vi "FTW-Test-Socket-Stress-PubSub.vi"() -> (0 "Test Result":errorcluster)   [LabVIEW 2014]
panel:
  in  "Test to Perform":T1(radio)=enum."12x100x10k"
  out "Progress":dbl(slide) scale=0.0..1.0
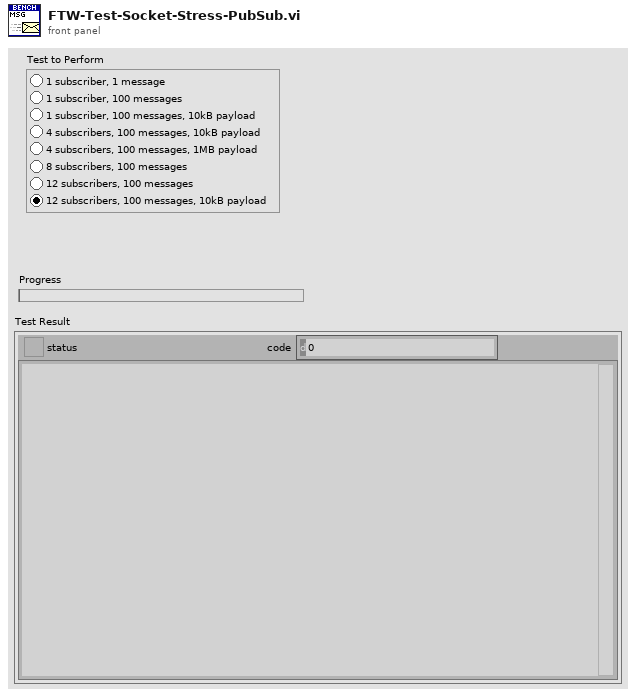
[diagram p1: front panel]
types:
  T1 = enum32{"1x1x0", "1x100x0", "1x100x10k", "4x100x10k", "4x100x1M", "8x100x0", "12x100x0", "12x100x10k"}
  T2 = typedef "FTW-Socket-Core-TransportScheme.ctl" = enum16{"TCP (tcp://)", "Inter-Process (ipc://)", "In-Process (inproc://)", "WebSocket (ws://)"}
  T3 = cluster{i32, "Bytes Recv'd":i32, "Messages Recv'd":i32}
  T4 = typedef "FTW-ERR-ExceptionType.ctl" = enum16{"OK", "Info", "Warning", "Error"}
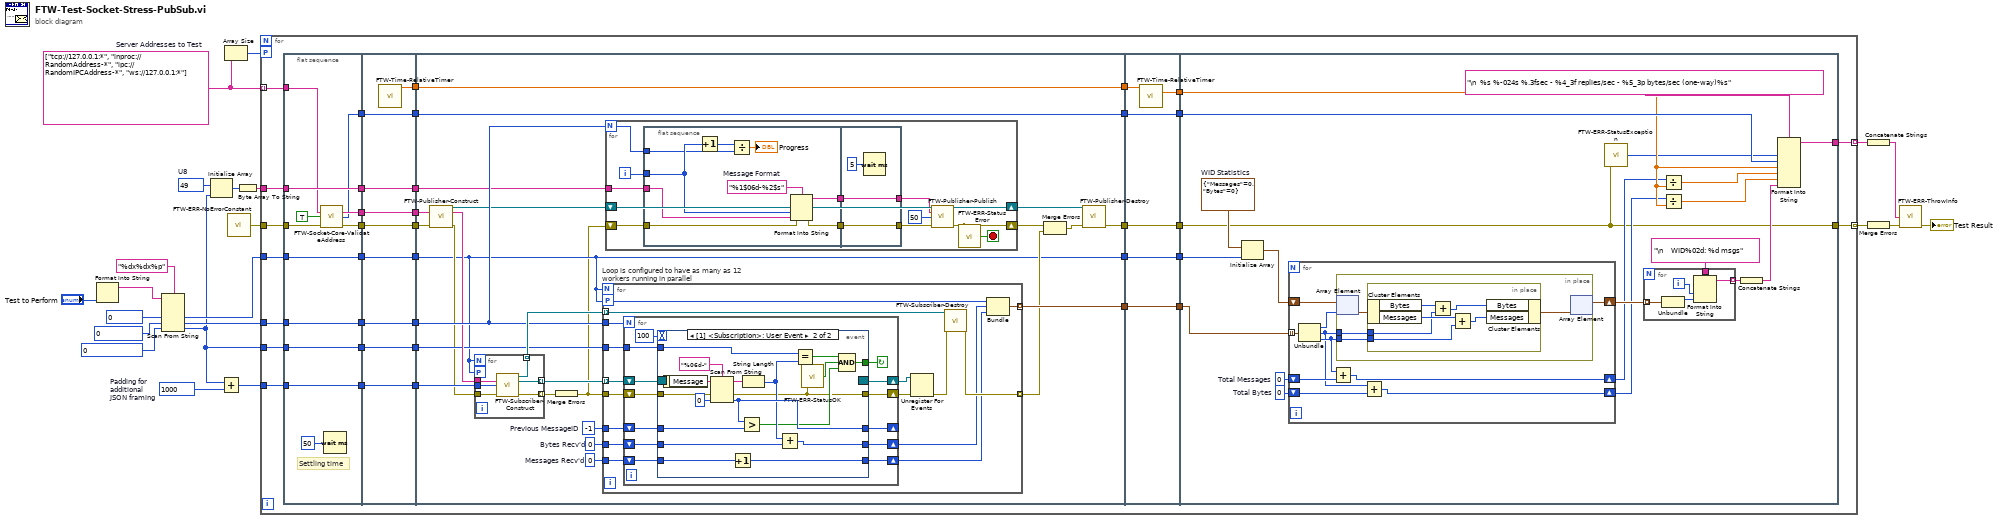
[diagram p0: block diagram]
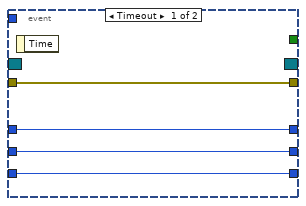
[diagram p2: hidden frame]
diagram:
  w2 = string[] ["tcp://127.0.0.1:*", "inproc://RandomAddress-*", "ipc://RandomIPCAddress-*", "ws://127.0.0.1:*"]  # Server Addresses to Test
  w19 = 1000  # Padding for additional JSON framing
  w22 = u8 49  # U8
  n1 = Format Into String("Test to Perform") -> (resulting string=w12:string)  [unwired: 3 in, 1 out]
  n2 = Scan From String(format string="%dx%dx%p", input string=w12, default 1=0, default 2=0, default 3=0) -> (output 1=w11:i32, output 2=w10:i32, output 3=w1:i32)  [unwired: 2 in, 3 out]
  n3 = Initialize Array(w22, w1) -> (w21:u8[])
  n4 = Add(x=w1, y=w19) -> (x+y=w18:i32)
  n5 = Array Size(array=w2) -> (size(s)=w3:i32)
  n6 = call "FTW-ERR-NoErrorConstant.vi"() -> ("no error"=w4:errorcluster)
  n7 = Byte Array To String(unsigned byte array=w21) -> (string=w20:string)
  n8 = for {
    tunnel: w2 -> [w51] mode=indexing
    tunnel: w11 -> [w50]
    tunnel: w10 -> [w48]
    tunnel: w4 -> [w47]
    tunnel: w20 -> [w40]
    tunnel: w18 -> [w34]
    tunnel: [w33] -> w9 mode=indexing
    tunnel: [w32] -> w7 mode=indexing
    workers-P: w3 -> [_]
    tunnel: w1 -> [w23]
    n9 = flat-sequence {
      tunnel: [w61] -> w58
      tunnel: [w63] -> w52
      tunnel: w47 -> [w62]
      tunnel: w48 -> [w67]
      tunnel: w50 -> [w68]
      tunnel: w51 -> [w64]
      tunnel: [w68] -> w45
      tunnel: [w67] -> w43
      tunnel: [w69] -> w41
      tunnel: w40 -> [w69]
      tunnel: [w66] -> w35
      tunnel: w34 -> [w66]
      tunnel: [w60] -> w30
      tunnel: [w59] -> w24
      tunnel: w23 -> [w59]
      tunnel: [w79] -> w57
      tunnel: [w74] -> w56
      tunnel: w58 -> [w79]
      tunnel: [w78] -> w53
      tunnel: w52 -> [w78]
      tunnel: [w77] -> w46
      tunnel: w45 -> [w77]
      tunnel: [w76] -> w44
      tunnel: w43 -> [w76]
      tunnel: [w75] -> w42
      tunnel: w41 -> [w75]
      tunnel: [w73] -> w36
      tunnel: w35 -> [w73]
      tunnel: [w72] -> w31
      tunnel: w30 -> [w72]
      tunnel: [w71] -> w25
      tunnel: w24 -> [w71]
      tunnel: [w93] -> w55
      tunnel: [w104] -> w54
      tunnel: [w103] -> w49
      tunnel: w44 -> [w96]
      tunnel: w46 -> [w81]
      tunnel: w57 -> [w102]
      tunnel: w56 -> [w104]
      tunnel: w53 -> [w92]
      tunnel: w42 -> [w88]
      tunnel: w36 -> [w89]
      tunnel: w31 -> [w87]
      tunnel: [w87] -> w28
      tunnel: [w81] -> w26
      tunnel: w25 -> [w83]
      tunnel: w55 -> [w192]
      tunnel: w54 -> [w190]
      tunnel: w49 -> [w191]
      tunnel: [w192] -> w39
      tunnel: [w189] -> w38
      tunnel: [w191] -> w37
      tunnel: [w188] -> w29
      tunnel: w28 -> [w188]
      tunnel: [w187] -> w27
      tunnel: w26 -> [w187]
      tunnel: w39 -> [w193]
      tunnel: w38 -> [w209]
      tunnel: w37 -> [w206]
      tunnel: [w193] -> w33
      tunnel: [w211] -> w32
      tunnel: w29 -> [w210]
      tunnel: w27 -> [w204]
      frame #0 {
        # "Settling time"
        n10 = call "FTW-Socket-Core-ValidateAddress.vi"("Address"=w64, "Allow wildcard replacement?"=TRUE, "error in"=w62) -> ("Sanitized Address"=w63:string, "Message Transport Scheme"=w60:T2, "error out"=w61:errorcluster)  [unwired: 10 in]
        n11 = Wait (ms)(milliseconds to wait=u32 50) -> ()  [unwired: 1 out]
      }
      frame #1 {
        n12 = call "FTW-Time-RelativeTimer.vi"() -> ("Current Uptime"=w74:dbl)  [unwired: 13 in, 2 out]
      }
      frame #2 {
        w84 = 0  # Messages Recv'd
        w86 = -1  # Previous MessageID
        w85 = 0  # Bytes Recv'd
        n13 = call "FTW-Publisher-Construct.vi"("Instance Inbox Address"=w92, "error in"=w102) -> ("FTW Publisher"=w91:refnum<data-value>, "Resolved Inbox Address"=w90:string, "error out"=w82:errorcluster)  [unwired: 11 in]
        n14 = for {
          N: w81 -> [_]
          workers-P: w81 -> [_]
          tunnel: w90 -> [w110]
          tunnel: w82 -> [w109]
          tunnel: [w108] -> w98 mode=indexing
          tunnel: [w107] -> w97 mode=indexing
          tunnel: [w106] -> w100 mode=indexing
          tunnel: w89 -> [w105]
          n15 = call "FTW-Subscriber-Construct.vi"("Publisher Address"=w110, "Receive Message Size Limit"=w105, "error in"=w109) -> ("FTW Subscriber"=w108:refnum<data-value>, "Subscription"=w107:refnum<event-registration>, "error out"=w106:errorcluster)  [unwired: 10 in]
        }
        n16 = Merge Errors(w100) -> (w80:errorcluster)
        n17 = for "Loop is configured to have as many as 12 workers running in parallel" {
          N: w81 -> [_]
          workers-P: w81 -> [w147]
          tunnel: [w151] -> w103 mode=indexing
          tunnel: [w146] -> w101 mode=indexing
          tunnel: w98 -> [w148] mode=indexing
          tunnel: w97 -> [w150] mode=indexing
          tunnel: w96 -> [w145]
          tunnel: w80 -> [w138]
          tunnel: w83 -> [w141]
          tunnel: w86 -> [w140]
          tunnel: w85 -> [w139]
          tunnel: w84 -> [w137]
          n18 = for {
            N: w145 -> [_]
            shift-right: [w162] -> w149
            shift-left: w150 -> [w164]
            shift-right: [w161] -> w144
            shift-left: w138 -> [w163]
            shift-right: [w156] -> w142
            shift-left: w139 -> [w158]
            shift-right: [w157] -> _
            shift-left: w140 -> [w159]
            tunnel: w141 -> [w160]
            shift-right: [w154] -> w136
            shift-left: w137 -> [w155]
            stop <- w153 continue-if-true
            n19 = event shown="[1] <Subscription>: User Event" {
              selector: w164 -> [_ _]
              dyn-events: [_ _] -> w162
              timeout: 100 -> [_ _]
              tunnel: [_ w171] -> w153
              tunnel: [w168 w172] -> w161
              tunnel: w163 -> [w168 w184]
              tunnel: w160 -> [_ w185]
              tunnel: w159 -> [w167 w182]
              tunnel: w158 -> [w166 w183]
              tunnel: [w167 w181] -> w157
              tunnel: [w166 w177] -> w156
              tunnel: w155 -> [w165 w178]
              tunnel: [w165 w176] -> w154
              event Timeout {
                n20 = event-data() -> ()  [unwired: 1 in, 1 out]
              }
              event User Event {
                n21 = event-data() -> ("Message"=w170:string)  [unwired: 1 in]
                n22 = Scan From String(format string="%06d-", input string=w170, error in=w184, default 1=0 ("default value 1")) -> (remaining string=w169:string, error out=w172:errorcluster, output 1=w181:i32)  [unwired: 1 in, 1 out]
                n23 = Increment(x=w178) -> (x+1=w176:i32)
                n24 = Greater?(x=w181, y=w182) -> (0:w174:bool)
                n25 = String Length(string=w169) -> (length=w179:i32)
                n26 = Add(x=w179, y=w183) -> (x+y=w177:i32)
                n27 = Equal?(x=w185, y=w179) -> (x = y?=w175:bool)
                n28 = call "FTW-ERR-StatusOK.vi"("error to check"=w172) -> ("Status OK?"=w173:bool)
                n29 = Compound Arithmetic op=AND(w175, w173, w174) -> (w171:bool)
              }
            }
          }
          n30 = Unregister For Events(event registration refnum=w149, error in=w144) -> (error out=w143:errorcluster)
          n31 = call "FTW-Subscriber-Destroy.vi"("FTW Subscriber"=w148, "error in"=w143) -> ("error out"=w146:errorcluster)  [unwired: 13 in]
          n32 = Bundle(w147, "Bytes Recv'd"=w142, "Messages Recv'd"=w136) -> (w151:T3)  [unwired: 1 in]
        }
        n33 = for {
          N: w96 -> [w113]
          shift-right: [w122] -> w99
          shift-left: w91 -> [w123]
          tunnel: w88 -> [w115]
          shift-right: [w120] -> w95
          shift-left: w80 -> [w117]
          i -> [w114]
          stop <- w119 stop-if-true
          n34 = flat-sequence {
            tunnel: w117 -> [w132]
            tunnel: [w131] -> w116
            tunnel: w115 -> [w130]
            tunnel: w114 -> [w126]
            tunnel: w113 -> [w125]
            tunnel: [w124] -> w111
            tunnel: [w135] -> w118
            tunnel: w116 -> [w135]
            tunnel: [w133] -> w112
            tunnel: w111 -> [w133]
            frame #0 {
              w129 = "%1$06d-%2$s"  # Message Format
              n35 = Increment(x=w126) -> (x+1=w127:i32)
              n36 = Divide(x=w127, y=w125) -> (x/y=→"Progress":dbl)
              n37 = Format Into String(format string=w129, error in=w132, w126, w130) -> (resulting string=w124:string, error out=w131:errorcluster)  [unwired: 1 in]
            }
            frame #1 {
              n38 = Wait (ms)(milliseconds to wait=u32 5) -> ()  [unwired: 1 out]
            }
          }
          n39 = call "FTW-Publisher-Publish.vi"("FTW Publisher"=w123, "Message"=w112, "Send Timeout"=50, "error in"=w118) -> ("FTW Publisher out"=w122:refnum<data-value>, "error out"=w120:errorcluster)  [unwired: 10 in]
          n40 = call "FTW-ERR-StatusError.vi"("error to check"=w120) -> ("Error?"=w119:bool)
        }
        n41 = Merge Errors(w95, w101) -> (w94:errorcluster)
        n42 = call "FTW-Publisher-Destroy.vi"("FTW Publisher"=w99, "error in"=w94) -> ("error out"=w93:errorcluster)  [unwired: 13 in]
      }
      frame #3 {
        n43 = call "FTW-Time-RelativeTimer.vi"("Previous Uptime"=w190) -> ("Elapsed Time"=w189:dbl)  [unwired: 12 in, 2 out]
      }
      frame #4 {
        w198 = 0  # Total Messages
        w197 = 0  # Total Bytes
        w205 = cluster{"Messages":i32, "Bytes":i32} {"Messages"=0, "Bytes"=0}  # WID Statistics
        n44 = Initialize Array(w205, w204) -> (w203:cluster{"Messages":i32, "Bytes":i32}[])
        n45 = for {
          tunnel: w206 -> [w227] mode=indexing
          shift-right: [w224] -> w202
          shift-left: w203 -> [w226]
          shift-right: [w220] -> w196
          shift-left: w198 -> [w223]
          shift-right: [w221] -> w195
          shift-left: w197 -> [w222]
          n46 = Unbundle(w227) -> (w225:i32, "Bytes Recv'd"=w218:i32, "Messages Recv'd"=w219:i32)
          n47 = Add(x=w219, y=w223) -> (x+y=w220:i32)
          n48 = in-place {
            in-place-border: w218 -> [w230]
            in-place-border: w219 -> [w229]
            n49 = in-place-array #1(w226, w225) -> (w231:cluster{"Messages":i32, "Bytes":i32})
            n50 = in-place {
              in-place-border: w230 -> [w233]
              in-place-border: w229 -> [w232]
              n51 = in-place-cluster #2(w231) -> ("Bytes"=w237:i32, "Messages"=w235:i32)
              n52 = Add(x=w237, y=w233) -> (x+y=w236:i32)
              n53 = Add(x=w235, y=w232) -> (x+y=w234:i32)
              n54 = in-place-cluster #2("Bytes"=w236, "Messages"=w234) -> (w228:cluster{"Messages":i32, "Bytes":i32})
            }
            n55 = in-place-array #1(w228) -> (w224:cluster{"Messages":i32, "Bytes":i32}[])  [unwired: 1 out]
          }
          n56 = Add(x=w218, y=w222) -> (x+y=w221:i32)
        }
        n57 = call "FTW-ERR-StatusException.vi"("error to check"=w193) -> ("Exception"=w194:T4)
        n58 = for {
          tunnel: w202 -> [w217] mode=indexing
          tunnel: [w215] -> w201 mode=indexing
          tunnel: "\n    WID%02d: %d msgs" ("format string") -> [w214]
          i -> [w216]
          n59 = Unbundle(w217) -> ("Messages"=w213:i32)  [unwired: 1 out]
          n60 = Format Into String(format string=w214, w216, w213) -> (resulting string=w215:string)  [unwired: 2 in, 1 out]
        }
        n61 = Divide(x=w196, y=w209) -> (x/y=w208:dbl)
        n62 = Divide(x=w195, y=w209) -> (x/y=w207:dbl)
        n63 = Concatenate Strings(w201) -> (w200:string)
        n64 = Format Into String(format string="\n  %s %-024s %.3fsec - %4_3f replies/sec - %5_3p bytes/sec (one-way)%s", w194, w210, w209, w208, w207, w200) -> (resulting string=w211:string)  [unwired: 2 in, 1 out]
      }
    }
  }
  n65 = Concatenate Strings(w7) -> (w6:string)
  n66 = Merge Errors(w9) -> (w5:errorcluster)
  n67 = call "FTW-ERR-ThrowInfo.vi"("Informational Message"=w6, "error in"=w5) -> ("error out"=→"Test Result":errorcluster)  [unwired: 13 in]
